vi "Q FPGA.vi"(8 "Error in":errorcluster, 9 "Timeout":i32=-1, 10 "Action":T2, 11 "Message FPGA in":T1) -> (0 "Error out":errorcluster, 1 "Timed out?":bool, 3 "Message FPGA out":T1)   [LabVIEW 2021]
uses:
  Typedefs/Q Action.ctl
  Typedefs/Message FPGA.ctl
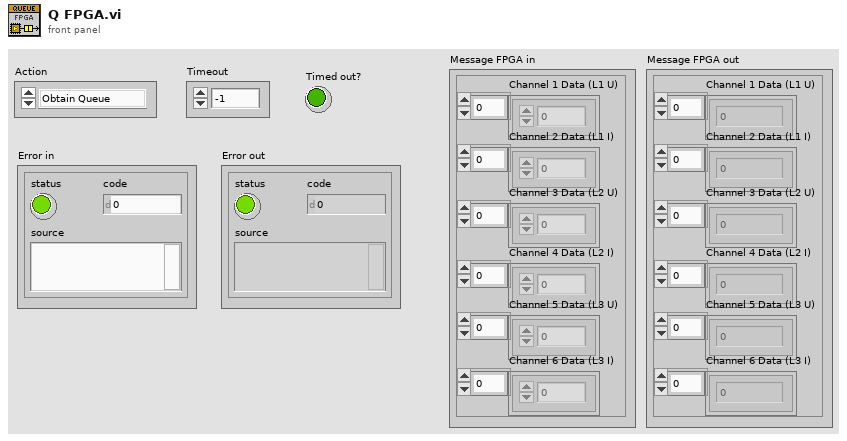
[diagram p1: front panel]
types:
  T1 = typedef "Message FPGA.ctl" = cluster{"Channel 1 Data (L1 U)":dbl[], "Channel 2 Data (L1 I)":dbl[], "Channel 3 Data (L2 U)":dbl[], "Channel 4 Data (L2 I)":dbl[], "Channel 5 Data (L3 U)":dbl[], "Channel 6 Data (L3 I)":dbl[]}
  T2 = typedef "Q Action.ctl" = enum16{"Obtain Queue", "Enqueue", "Dequeue", "Close"}
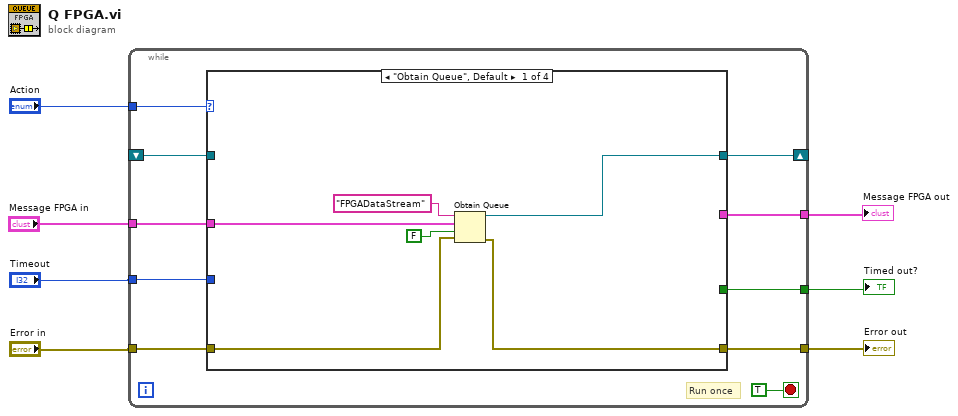
[diagram p0: block diagram]
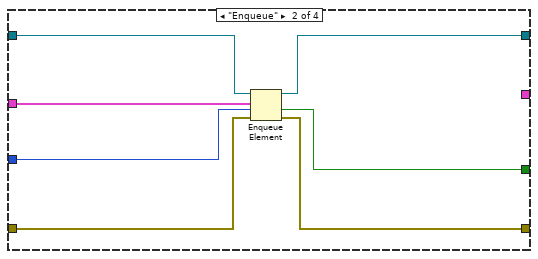
[diagram p2: hidden frame]
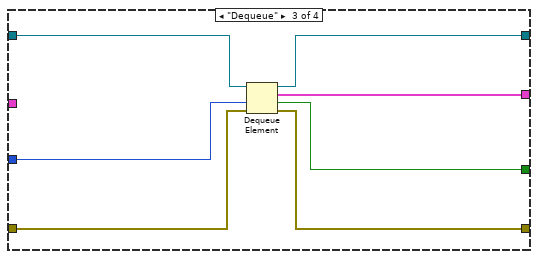
[diagram p3: hidden frame]
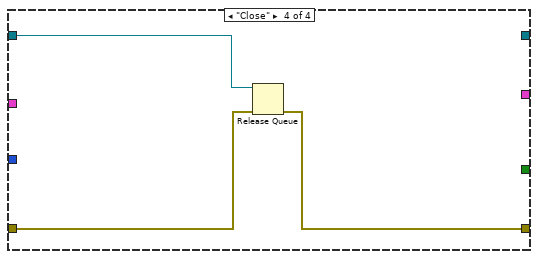
[diagram p4: hidden frame]
diagram:
  n1 = while {
    tunnel: "Action" -> [w16]
    shift-right: [w15] -> _
    shift-left: _ -> [w14]
    tunnel: "Message FPGA in" -> [w11]
    tunnel: "Timeout" -> [w12]
    tunnel: "Error in" -> [w13]
    tunnel: [w10] -> w1
    tunnel: [w9] -> w4
    tunnel: [w8] -> w3
    stop <- TRUE stop-if-true
    # "Run once"
    n2 = case shown="\"Obtain Queue\", Default" w16 {
      tunnel: [w23 w29 w36 _] -> w15
      tunnel: w14 -> [_ w30 w37 w40]
      tunnel: w13 -> [w21 w26 w32 w39]
      tunnel: w12 -> [_ w27 w33 _]
      tunnel: w11 -> [w20 w28 _ _]
      tunnel: [_ _ w34 _] -> w10
      tunnel: [w22 w25 w31 w38] -> w9
      tunnel: [_ w24 w35 _] -> w8
      frame "Obtain Queue", Default {
        n3 = Obtain Queue(name (unnamed)="FPGADataStream", element data type=w20, create if not found? (T)=FALSE, error in (no error)=w21) -> (queue out=w23:refnum<queue>, error out=w22:errorcluster)  [unwired: 1 in, 1 out]
      }
      frame "Enqueue" {
        n4 = Enqueue Element(queue=w30, element=w28, timeout in ms (-1)=w27, error in (no error)=w26) -> (queue out=w29:refnum<queue>, timed out?=w24:bool, error out=w25:errorcluster)
      }
      frame "Dequeue" {
        n5 = Dequeue Element(queue=w37, timeout in ms (-1)=w33, error in (no error)=w32) -> (queue out=w36:refnum<queue>, element=w34:T1, timed out?=w35:bool, error out=w31:errorcluster)
      }
      frame "Close" {
        n6 = Release Queue(queue=w40, error in (no error)=w39) -> (error out=w38:errorcluster)  [unwired: 1 in, 2 out]
      }
    }
  }
  "Timed out?" <- w3
  "Error out" <- w4
  "Message FPGA out" <- w1
